vi "Drop RPC Methods in SyncMethod Event Structure.vi"(8 "error in (no error)":errorcluster, 10 "dynamic member VIs":refnum<vi>[](array[refnum]), 11 "Server class in":refnum<vi>) -> (0 "error out":errorcluster, 3 "Server class out":refnum<vi>)   [LabVIEW 2019, in "gRPC Template Creation Utility.lvlib"]
uses:
  gRPC Template Creation Utility.lvlib
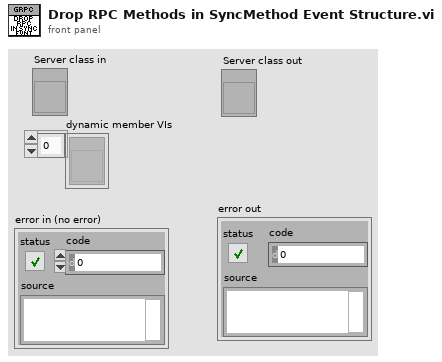
[diagram p1: front panel]
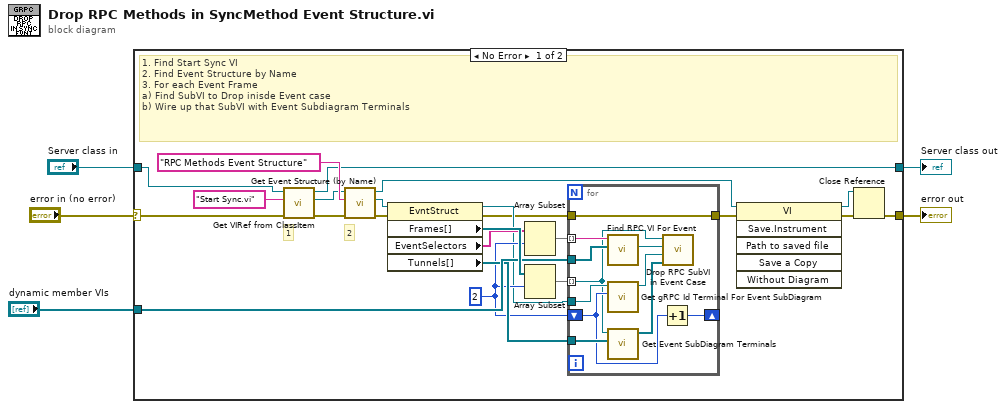
[diagram p0: block diagram]
diagram:
  n1 = case shown="No Error" "error in (no error)" {
    selector: "error in (no error)" -> [w24 w41]
    tunnel: [w6 w41] -> w4
    tunnel: "Server class in" -> [w27 w40]
    tunnel: [w13 w40] -> w2
    tunnel: "dynamic member VIs" -> [w17 _]
    frame No Error {
      w15 = 2 ("index")
      # "2"
      # "1"
      # "1. Find Start Sync VI\n2. Find Event Structure by Name\n3. For each Event Frame\na) Find SubVI to Drop inisde Event case\nb) Wire up that SubVI with Event Subdiagram Terminals"
      n2 = call "Get VIRef from ClassItem.vi"("error in (no error)"=w24, "Item Name"="Start Sync.vi", "LVClassLibrary in"=w27) -> ("error out"=w23:errorcluster, "VIref out"=w25:refnum<vi>, "LVClassLibrary out"=w13:refnum<vi>)  [unwired: 5 in, 1 out]
      n3 = call "Get Event Structure (by Name).vi"("error in (no error)"=w23, "Label"="RPC Methods Event Structure", "Owner VI in"=w25) -> ("error out"=w12:errorcluster, "Event Structure ref out"=w22:refnum<vi>, "Owner VI out"=w9:refnum<vi>)  [unwired: 5 in, 1 out]
      n4 = property class="EvntStruct"(reference=w22, error in=w12) -> (reference out=w14:refnum<vi>, error out=w11:errorcluster, "Frames[]"=w21:refnum<vi>[], "EventSelectors"=w20:string[], "Tunnels[]"=w16:refnum<vi>[])
      n5 = Array Subset(array=w20, index=w15) -> (w18:string[])  [unwired: 1 in]
      n6 = Array Subset(array=w21, index=w15) -> (w19:refnum<vi>[])  [unwired: 1 in]
      n7 = for {
        tunnel: w19 -> [w30] mode=indexing
        tunnel: w18 -> [w39] mode=indexing
        tunnel: w17 -> [w38]
        tunnel: w16 -> [w37]
        shift-right: [w36] -> _
        shift-left: w15 -> [w35]
        tunnel: w14 -> [w34]
        tunnel: w11 -> [w29]
        tunnel: [w29] -> w10
        n8 = call "Find RPC VI For Event.vi"("RPC VIs in"=w38, "input event string"=w39) -> ("RPC VI out"=w32:refnum<vi>)  [unwired: 8 in, 1 out]
        n9 = call "Get gRPC Id Terminal For Event SubDiagram.vi"("Frame Index in"=w35, "Event Structure ref in"=w34) -> ("Term Refnum"=w33:refnum<vi>)  [unwired: 9 in]
        n10 = call "Get Event SubDiagram Terminals.vi"("All Event Structure Tunnels"=w37, "Event Subdiagram in"=w30) -> ("SubDiagram Terminals out"=w31:refnum<vi>[])  [unwired: 9 in]
        n11 = Increment(x=w35) -> (x+1=w36:i32)
        n12 = call "Drop RPC SubVI in Event Case.vi"("SubDiagram Terminals in"=w31, "gRPC Id EventData Terminal Refnum in"=w33, "RPC VI in"=w32, "Subdiagram Refnum in"=w30) -> ()  [unwired: 8 in]
      }
      n13 = invoke class="VI" method="Save.Instrument"(reference=w9, error in=w10) -> (reference out=w8:refnum<vi>, error out=w7:errorcluster)  [unwired: 4 in, 4 out]
      n14 = Close Reference(reference=w8, error in (no error)=w7) -> (error out=w6:errorcluster)
    }
    frame Error {
    }
  }
  "error out" <- w4
  "Server class out" <- w2
